vi "Overlay Results (Concentric).vi"(5 "Setup":T2, 6 "Scan Direction":u32(ring) items=["Counter-Clockwise", "Clockwise"], 7 "ROI Descriptor":T1 {"Contours"."Type" items=["No Selection", "Point", "Line", "Rectangle", "Oval", "Polygon", "Free", "Annulus", "Unused2", "Unused3", "Broken Line", "Free Hand Line", "Rotated Rectangle"]}, 8 "Line Radius":i32[](array[numeric]), 9 "All Edges Found":cluster{"X":sgl, "Y":sgl}[](array[cluster])=[{"X"=27.450102, "Y"=144.0}, {"X"=70.80146, "Y"=144.0}, {"X"=114.11963, "Y"=144.0}, {"X"=158.60345, "Y"=144.0}, {"X"=202.3678, "Y"=144.0}, {"X"=246.04292, "Y"=144.0}, {"X"=291.42203, "Y"=144.0}, {"X"=336.54822, "Y"=144.0}, {"X"=379.2348, "Y"=144.0}, {"X"=425.02194, "Y"=144.0}, {"X"=467.72144, "Y"=144.0}, {"X"=26.88918, "Y"=210.0}, {"X"=70.6191, "Y"=210.0}, {"X"=115.31038, "Y"=210.0}, {"X"=159.03351, "Y"=210.0}, {"X"=202.2118, "Y"=210.0}, {"X"=247.37573, "Y"=210.0}, {"X"=292.001, "Y"=210.0}, {"X"=336.55954, "Y"=210.0}, {"X"=379.72208, "Y"=210.0}, {"X"=424.86005, "Y"=210.0}, {"X"=468.8485, "Y"=210.0}, {"X"=26.897532, "Y"=309.0}, {"X"=70.88008, "Y"=309.0}, {"X"=114.93419, "Y"=309.0}, {"X"=159.13483, "Y"=309.0}, {"X"=203.12064, "Y"=309.0}, {"X"=247.9202, "Y"=309.0}, {"X"=291.07425, "Y"=309.0}, {"X"=335.25354, "Y"=309.0}, {"X"=378.88284, "Y"=309.0}, {"X"=424.06085, "Y"=309.0}, {"X"=469.80658, "Y"=309.0}] {"Y" format="%.2f"; "X" format="%.2f"}, 10 "Line Coordinates":T3 {"Point2"."Y" format="%.2f"; "Point2"."X" format="%.2f"; "Point1"."Y" format="%.2f"; "Point1"."X" format="%.2f"}, 11 "Image In":T4) -> (3 "Image Out":T4)   [LabVIEW 2020]
uses:
  IMAQ Image.ctl
panel:
  in  "Result Color":u32(colorbox)=16711680
  in  "Edge Locations Color":u32(colorbox)=16776960
  in  "Search Lines Color":u32(colorbox)=26367
  in  "Search Area Color":u32(colorbox)=65280
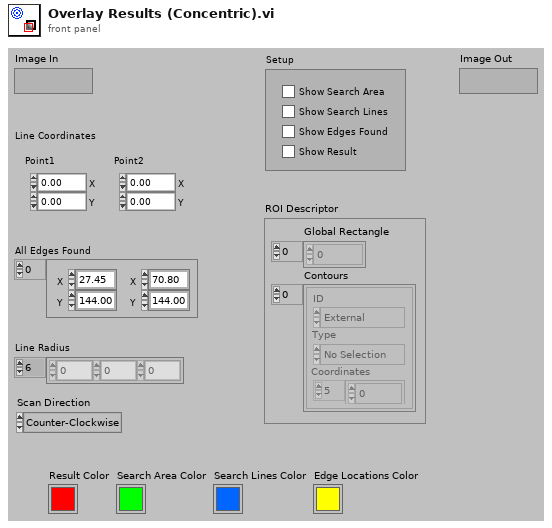
[diagram p1: front panel]
types:
  T1 = cluster{"Global Rectangle":i32[], "Contours":cluster{"ID":enum32{"External", "Internal"}, "Type":u32, "Coordinates":i32[]}[]}
  T2 = cluster{"Show Search Area":bool, "Show Search Lines":bool, "Show Edges Found":bool, "Show Result":bool}
  T3 = cluster{"Point1":cluster{"X":sgl, "Y":sgl}, "Point2":cluster{"X":sgl, "Y":sgl}}
  T4 = typedef "IMAQ Image.ctl" = refnum<image>
  T5 = typedef "IMAQ Circle" = cluster{"Center X":i32, "Center Y":i32, "Inner Radius":i32, "Outer Radius":i32, "Start Angle":dbl, "End Angle":dbl}
  T6 = cluster{"[0]":i32, "[1]":i32, "[2]":i32, "[3]":i32}
  T7 = cluster{"[0]":sgl, "[1]":sgl, "[2]":sgl, "[3]":sgl}
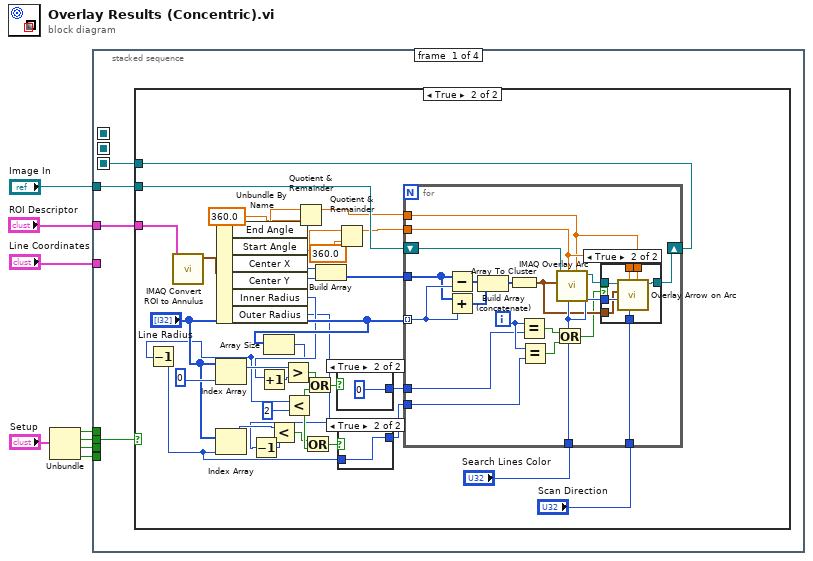
[diagram p0: block diagram]
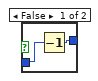
[diagram p3: hidden frame]
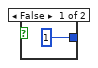
[diagram p4: hidden frame]
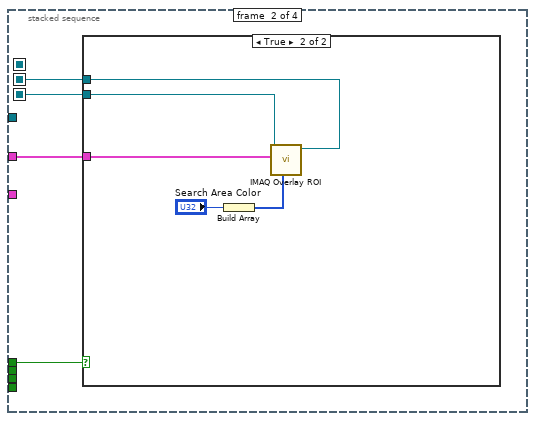
[diagram p6: hidden frame]
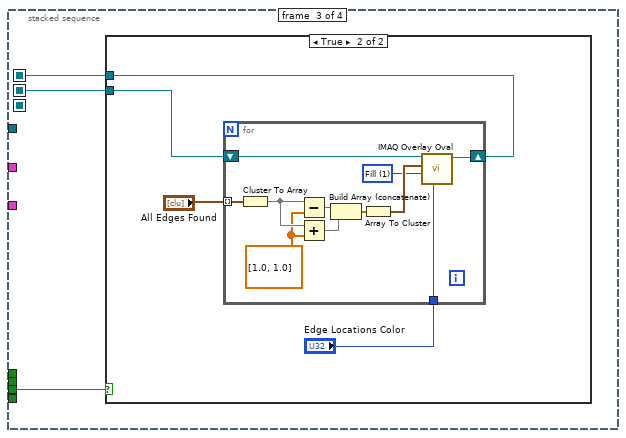
[diagram p8: hidden frame]
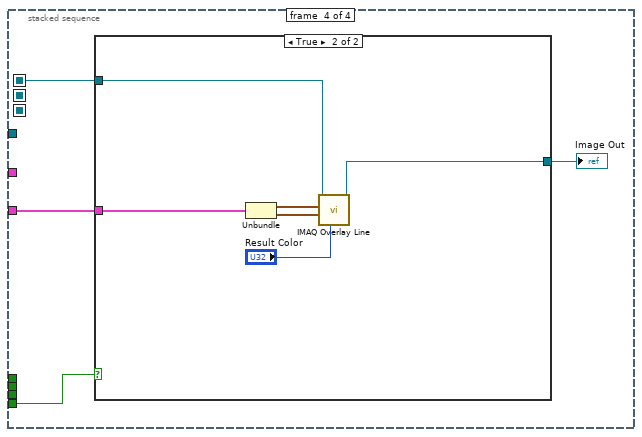
[diagram p10: hidden frame]
diagram:
  n1 = Unbundle("Setup") -> ("Show Search Area"=w4:bool, "Show Search Lines"=w5:bool, "Show Edges Found"=w3:bool, "Show Result"=w2:bool)
  n2 = stacked-sequence {
    seq-local: [_ _ w91 _] -> [_ _ _ w111]
    seq-local: [w11 _ _ _] -> [_ w81 _ _]
    seq-local: [_ w82 _ _] -> [_ _ w90 _]
    tunnel: "Image In" -> [w12 _ _ _]
    tunnel: "Line Coordinates" -> [_ _ _ w110]
    tunnel: w5 -> [w10 _ _ _]
    tunnel: w4 -> [_ w80 _ _]
    tunnel: w3 -> [_ _ w89 _]
    tunnel: w2 -> [_ _ _ w109]
    tunnel: "ROI Descriptor" -> [w9 w79 _ _]
    frame #0 {
      n3 = case shown="True" w10 {
        tunnel: w12 -> [w13 w46]
        tunnel: [w13 w45] -> w11
        tunnel: w9 -> [_ w40]
        frame False {
        }
        frame True {
          n4 = call "IMAQ Convert ROI to Annulus"("ROI Descriptor"=w40) -> ("Annulus"=w43:T5)  [unwired: 1 in, 8 out]
          n5 = Index Array(array="Line Radius", index=0 ("Index")) -> (element=w36:i32)
          n6 = Unbundle By Name(w43) -> ("End Angle"=w20:dbl, "Start Angle"=w15:dbl, "Center X"=w42:i32, "Center Y"=w41:i32, "Inner Radius"=w35:i32, "Outer Radius"=w23:i32)
          n7 = Decrement(x=w23) -> (x-1=w24:i32)
          n8 = Increment(x=w35) -> (x+1=w34:i32)
          n9 = Array Size(array="Line Radius") -> (size(s)=w33:i32)
          n10 = Decrement(x=w33) -> (x-1=w22:i32)
          n11 = Index Array(array="Line Radius", index=w22) -> (element=w25:i32)
          n12 = Less?(x=w25, y=w24) -> (x < y?=w26:bool)
          n13 = Greater?(x=w36, y=w34) -> (0:w29:bool)
          n14 = Less?(x=w33, y=2) -> (x < y?=w30:bool)
          n15 = Quotient & Remainder(x=w20, y=360.0) -> (x-y*floor(x/y)=w18:dbl)  [unwired: 1 out]
          n16 = Or(x=w26, y=w30) -> (x .or. y?=w27:bool)
          n17 = Or(x=w29, y=w30) -> (x .or. y?=w31:bool)
          n18 = Build Array(w42, w41) -> (w17:i32[])
          n19 = Quotient & Remainder(x=w15, y=360.0) -> (x-y*floor(x/y)=w16:dbl)  [unwired: 1 out]
          n20 = case shown="True" w31 {
            tunnel: [1 0] -> w28
            frame False {
            }
            frame True {
            }
          }
          n21 = case shown="True" w27 {
            tunnel: w22 -> [w47 w49]
            tunnel: [w48 w49] -> w21
            frame False {
              n22 = Decrement(x=w47) -> (x-1=w48:i32)
            }
            frame True {
            }
          }
          n23 = for {
            shift-right: [w63] -> w45
            shift-left: w46 -> [w70]
            tunnel: "Search Lines Color" -> [w62]
            tunnel: "Line Radius" -> [w69] mode=indexing
            tunnel: w17 -> [w65]
            tunnel: w16 -> [w59]
            tunnel: w18 -> [w58]
            tunnel: "Scan Direction" -> [w60]
            tunnel: w28 -> [w53]
            tunnel: w21 -> [w52]
            i -> [w54]
            n24 = Subtract(x=w65, y=w69) -> (x-y=w68:i32[])
            n25 = Add(x=w65, y=w69) -> (x+y=w67:i32[])
            n26 = Build Array (concatenate)(w68, w67) -> (w66:i32[])
            n27 = Array To Cluster(array=w66) -> (cluster=w61:T6)
            n28 = Equal?(x=w54, y=w53) -> (x = y?=w56:bool)
            n29 = Equal?(x=w54, y=w52) -> (x = y?=w55:bool)
            n30 = Or(x=w56, y=w55) -> (x .or. y?=w57:bool)
            n31 = call "IMAQ Overlay Arc"("End Angle (degrees)"=w58, "Color"=w62, "Start Angle (degrees)"=w59, "Bounding Rectangle"=w61, "Image"=w70) -> ("Image Out"=w64:T4)  [unwired: 3 in, 3 out]
            n32 = case shown="True" w57 {
              tunnel: w64 -> [w71 w72]
              tunnel: [w71 w78] -> w63
              tunnel: w62 -> [_ w77]
              tunnel: w61 -> [_ w76]
              tunnel: w60 -> [_ w75]
              tunnel: w59 -> [_ w74]
              tunnel: w58 -> [_ w73]
              frame False {
              }
              frame True {
                n33 = call "Overlay Arrow on Arc.vi"("End Angle (degrees)"=w73, "Scan Direction"=w75, "Start Angle (degrees)"=w74, "Color"=w77, "Bounding Rectangle"=w76, "Image"=w72) -> ("Image Out"=w78:T4)  [unwired: 1 in, 4 out]
              }
            }
          }
        }
      }
    }
    frame #1 {
      n34 = case shown="True" w80 {
        tunnel: [w83 w87] -> w82
        tunnel: w81 -> [w83 w88]
        tunnel: w79 -> [_ w84]
        frame False {
        }
        frame True {
          n35 = Build Array("Search Area Color") -> (w85:u32[])
          n36 = call "IMAQ Overlay ROI"("Colors (Green)"=w85, "ROI Descriptor"=w84, "Image"=w88) -> ("Image Out"=w87:T4)  [unwired: 3 in, 5 out]
        }
      }
    }
    frame #2 {
      n37 = case shown="True" w89 {
        tunnel: [w92 w96] -> w91
        tunnel: w90 -> [w92 w94]
        frame False {
        }
        frame True {
          n38 = for {
            shift-right: [w106] -> w96
            shift-left: w94 -> [w107]
            tunnel: "All Edges Found" -> [w105] mode=indexing
            tunnel: "Edge Locations Color" -> [w98]
            w97 = u32 1 items=["Frame", "Fill"] ("Drawing Mode (Frame)")
            w99 = sgl[] [1.0, 1.0] ("y")
            n39 = Cluster To Array(cluster=w105) -> (array=w104:sgl[])
            n40 = Subtract(x=w104, y=w99) -> (x-y=w103:sgl[])
            n41 = Add(x=w104, y=w99) -> (x+y=w102:sgl[])
            n42 = Build Array (concatenate)(w103, w102) -> (w101:sgl[])
            n43 = Array To Cluster(array=w101) -> (cluster=w100:T7)
            n44 = call "IMAQ Overlay Oval"("Color"=w98, "Drawing Mode (Frame)"=w97, "Bounding Rectangle"=w100, "Image"=w107) -> ("Image Out"=w106:T4)  [unwired: 2 in, 5 out]
          }
        }
      }
    }
    frame #3 {
      n45 = case shown="True" w109 {
        tunnel: w111 -> [w112 w114]
        tunnel: w110 -> [_ w118]
        tunnel: [w112 w115] -> w108
        frame False {
        }
        frame True {
          n46 = Unbundle(w118) -> ("Point1"=w113:cluster{"X":sgl, "Y":sgl}, "Point2"=w117:cluster{"X":sgl, "Y":sgl})
          n47 = call "IMAQ Overlay Line"("Color"="Result Color", "End Point"=w117, "Start Point"=w113, "Image"=w114) -> ("Image Out"=w115:T4)  [unwired: 2 in, 5 out]
        }
      }
      "Image Out" <- w108
    }
  }
